vi "Begin.vi"(11 "Image Size":T1=enum."160x120") -> (0 "error out":errorcluster)   [LabVIEW 2012]
doc: "Called before other user functions, this VI is expected to open initial I/O refnums, load in file data, and do all program initialization. Notice that the <B>error out</B> terminal is simply used for data flow. Wiring it to other structures or subVIs ensures that this VI runs first."
uses:
  <vilib>/Rock Robotics/WPI/Camera/WPI_CameraImageSize.ctl
  <vilib>/Rock Robotics/SystemInterfaces/DIO/FPGA_DIOChannel.ctl
  <vilib>/Rock Robotics/WPI/CAN/Jaguar/SubVIs/WPI_CANJaguar_ControlMode.ctl
  <vilib>/Rock Robotics/WPI/Solenoid/WPI_SolenoidChannel.ctl
  <vilib>/Rock Robotics/SystemInterfaces/DIO/FPGA_DIORelayChannel.ctl
  <vilib>/Rock Robotics/WPI/Joystick/WPI_JoystickDeviceEnum.ctl
  <vilib>/Rock Robotics/SystemInterfaces/DIO/FPGA_DIOPWMChannel.ctl
  <vilib>/Rock Robotics/WPI/SafetyOutput/WPI_SafetyOutputConfigMenu.ctl
  <vilib>/Rock Robotics/WPI/Camera/WPI_CameraWhite Balance Values.ctl
  <vilib>/Rock Robotics/WPI/Camera/WPI_CameraExposure Values.ctl
  <vilib>/Rock Robotics/WPI/Camera/WPI_CameraFrameRate.ctl
  <vilib>/Rock Robotics/WPI/DriverStation/WPI_DriverStationRobotMode2.ctl
  <vilib>/Rock Robotics/WPI/MotorControl/WPI_MotorControlOpenCANJaguar.vi
  <vilib>/Rock Robotics/WPI/Solenoid/WPI_SolenoidOpenSingle.vi
  <vilib>/Rock Robotics/WPI/RobotDrive/WPI_RobotDriveOpen2MotorWithJaguar.vi
  Robot Global Data.vi
  <vilib>/Rock Robotics/WPI/Compressor/WPI_CompressorGetSetRefNum.vi
  <vilib>/Rock Robotics/WPI/CAN/Jaguar/SubVIs/WPI_CANJaguar_SpeedReference.ctl
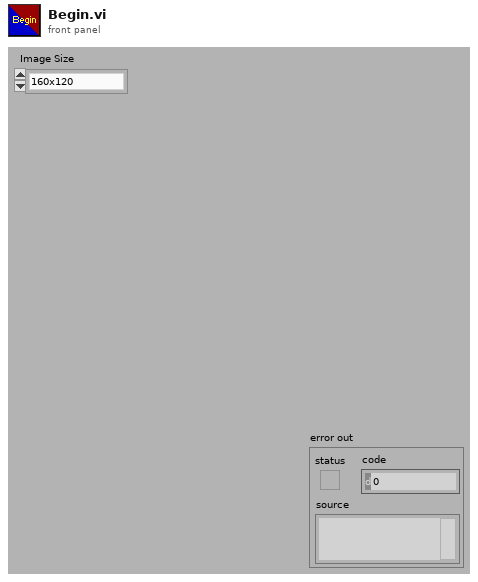
[diagram p1: front panel]
types:
  T1 = typedef "WPI_CameraImageSize.ctl" = enum16{"640x480", "320x240", "160x120"}
  T2 = typedef "WPI_DriverStationRobotMode2.ctl" = enum16{"Autonomous Disabled", "Autonomous Enabled", "Teleop Disabled", "Teleop Enabled", "Timeout", "Finish", "Test Disabled", "Test Enabled"}
  T3 = typedef "WPI_CameraFrameRate.ctl" = u32
  T4 = typedef "WPI_CameraExposure Values.ctl" = enum16{"Auto", "Flicker-free 50 Hz", "Flicker-free 60 Hz", "Hold current"}
  T5 = typedef "WPI_CameraWhite Balance Values.ctl" = enum16{"Auto", "Fixed indoor", "Fixed outdoor 1", "Fixed outdoor 2", "Fixed fluorescent 1", "Fixed fluorescent 2", "Hold current"}
  T6 = typedef "WPI_SafetyOutputConfigMenu.ctl" = enum16{"Enable", "Disable"}
  T7 = typedef "FPGA_DIOPWMChannel.ctl" = enum8{"PWM 1", "PWM 2", "PWM 3", "PWM 4", "PWM 5", "PWM 6", "PWM 7", "PWM 8", "PWM 9", "PWM 10", "Invalid"}
  T8 = typedef "WPI_JoystickDeviceEnum.ctl" = enum16{"USB 1", "USB 2", "USB 3", "USB 4", "Kinect 1", "Kinect 2"}
  T9 = typedef "FPGA_DIORelayChannel.ctl" = enum8{"Relay 1", "Relay 2", "Relay 3", "Relay 4", "Relay 5", "Relay 6", "Relay 7", "Relay 8", "Invalid"}
  T10 = typedef "WPI_SolenoidChannel.ctl" = enum8{"Solenoid 1", "Solenoid 2", "Solenoid 3", "Solenoid 4", "Solenoid 5", "Solenoid 6", "Solenoid 7", "Solenoid 8", "Invalid"}
  T11 = typedef "FPGA_DIOChannel.ctl" = enum8{"DIO 1", "DIO 2", "DIO 3", "DIO 4", "DIO 5", "DIO 6", "DIO 7", "DIO 8", "DIO 9", "DIO 10", "DIO 11", "DIO 12", "DIO 13", "DIO 14", "Invalid"}
  T12 = typedef "WPI_CANJaguar_ControlMode.ctl" = enum8{"Percent VBus", "Current", "Speed", "Position", "Voltage"}
  T13 = typedef "WPI_MotorControlDeviceRef.ctl" = cluster{"DeviceStatus":errorcluster, "Type":enum16{"PWM", "CAN"}, "PWM":cluster{"Digital Module":T14, "PWM Channel":T7, "DeadBand":T15}, "CAN":cluster{"Device Number":u8, "Control Mode":T12, "Semaphore":T16, "Max Vout":dbl}, "Invert":bool, "TransformRef":T17, "InvTransformRef":T17}
  T14 = typedef "FPGA_TypedefDigitalModule.ctl" = enum16{"Digital Module 1", "Digital Module 2"}
  T15 = typedef "WPI_PWMDeadband.ctl" = cluster{"Name":string, "maxPositivePwm":i32, "minPositivePwm":i32, "centerPwm":i32, "maxNegativePwm":i32, "minNegativePwm":i32, "angularRange":u16}
  T16 = typedef "Semaphore RefNum" = refnum<k1>
  T17 = typedef "WPI_PWMTransform_ConPane.ctl" = refnum<vi>
  T18 = typedef "WPI_CANJaguar_SpeedReference.ctl" = u8
  T19 = typedef "WPI_DigitalInputDevRef.ctl" = cluster{"DevStatus":errorcluster, "DIO Channel":T11, "Digital Module":T14}
  T20 = typedef "WPI_DigitalOutputDevRef.ctl" = cluster{"Digital Module":T14, "DIO Channel":T11, "DevStatus":errorcluster}
  T21 = typedef "WPI_JoystickDevRef.ctl" = cluster{"Device":T8}
  T22 = typedef "WPI_CompressorDevRef.ctl" = cluster{"DevStatus":errorcluster, "DigitalInputDevRef":T19, "RelayDevRef":T23}
  T23 = typedef "WPI_RelayDevRef.ctl" = cluster{"DevStatus":errorcluster, "Relay Channel":T9, "Digital Module":T14, "Relay Direction":T24}
  T24 = typedef "WPI_RelayDirection.ctl" = enum16{"Both directions", "Forward only", "Reverse only"}
  T25 = typedef "WPI_SolenoidDevRef.ctl" = cluster{"DevStatus":errorcluster, "Solenoid Module":T26, "Forward Solenoid Channel":T10, "Reverse Solenoid Channel":T10}
  T26 = typedef "FPGA_TypedefSolenoidModule.ctl" = enum16{"Solenoid Module 1", "Solenoid Module 2"}
  T27 = typedef "WPI_CameraDevRef.ctl" = cluster{"Camera Address":string, "CameraStatus":errorcluster, "Acquire Image Notifier":refnum<notifier>}
  T28 = typedef "WPI_RobotDriveDevRef.ctl" = cluster{"DevStatus":errorcluster, "Motors[]":T13[], "Square Inputs":bool, "Max Output":dbl, "Isochronous":bool}
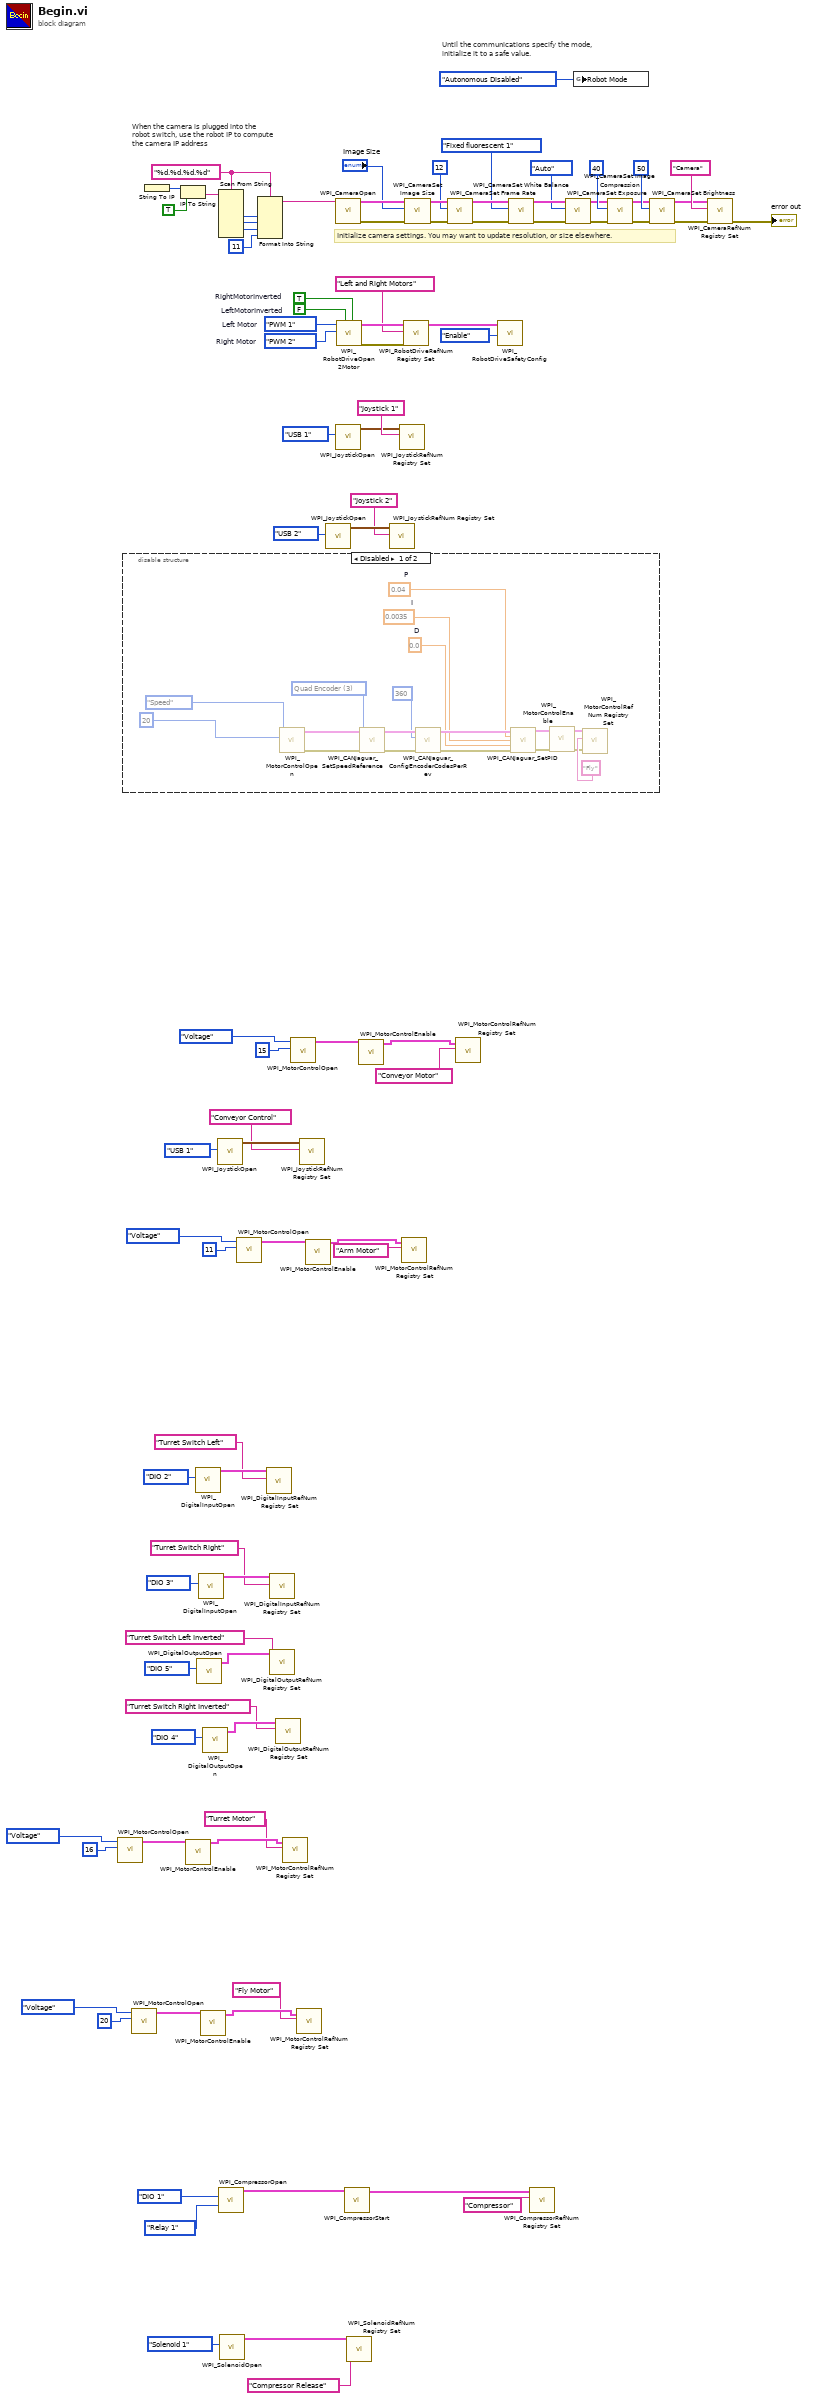
[diagram p0: block diagram]
diagram:
  w4 = "%d.%d.%d.%d" ("format string")
  w35 = FPGA_DIOPWMChannel."PWM 2"  # Right Motor
  w36 = FPGA_DIOPWMChannel."PWM 1"  # Left Motor
  w40 = FALSE  # LeftMotorInverted
  w41 = TRUE  # RightMotorInverted
  # "Until the communications specify the mode,\ninitialize it to a safe value."
  # "When the camera is plugged into the\nrobot switch, use the robot IP to compute\nthe camera IP address"
  # "Initialize camera settings. You may want to update resolution, or size elsewhere."
  n1 = call-poly <vilib>:"WPI_MotorControlOpen.vi"("Device Number"=u8 16, "Control Mode"=WPI_CANJaguar_ControlMode."Voltage") -> ("MotorControlDeviceRef"=w63:T13)  [unwired: 8 in, 1 out]
  n2 = disable-structure shown="Disabled" {
    frame Disabled {
      w93 = 0.0  # D
      w94 = 0.0035  # I
      w95 = 0.04  # P
      w99 = T18 3 items=["Encoder"=0, "Inv Encoder"=2, "Quad Encoder"=3, "None"=255] ("Speed Reference")
      n3 = call-poly <vilib>:"WPI_MotorControlOpen.vi"("Device Number"=u8 20, "Control Mode"=WPI_CANJaguar_ControlMode."Speed") -> ("error out"=w103:errorcluster, "MotorControlDeviceRef"=w102:T13)  [unwired: 8 in]
      n4 = call <vilib>:"WPI_CANJaguar_SetSpeedReference.vi"("error in (no error)"=w103, "Speed Reference"=w99, "CAN Jaguar Ref"=w102) -> ("error out"=w101:errorcluster, "CAN Jaguar Ref Out"=w100:T13)  [unwired: 7 in]
      n5 = call <vilib>:"WPI_CANJaguar_ConfigEncoderCodesPerRev.vi"("error in (no error)"=w101, "Encoder Codes Per Rev"=u16 360, "CAN Jaguar Ref"=w100) -> ("error out"=w96:errorcluster, "CAN Jaguar Ref Out"=w97:T13)  [unwired: 7 in]
      n6 = call <vilib>:"WPI_CANJaguar_SetPID.vi"("CAN Jaguar Ref"=w97, "P"=w95, "I"=w94, "D"=w93, "error in (no error)"=w96) -> ("CAN Jaguar Ref Out"=w92:T13, "error out"=w91:errorcluster)  [unwired: 9 in]
      n7 = call <vilib>:"WPI_MotorControlEnable.vi"("error in (no error)"=w91, "CAN Jaguar Ref"=w92) -> ("error out"=w104:errorcluster, "CAN Jaguar Ref Out"=w106:T13)  [unwired: 8 in]
      n8 = call <vilib>:"WPI_MotorControlRefNum Registry Set.vi"("error in (no error)"=w104, "refnum name"="Fly", "MotorControlDevRef"=w106) -> ()  [unwired: 7 in, 2 out]
    }
    frame Enabled {
    }
  }
  n9 = call-poly <vilib>:"WPI_MotorControlOpen.vi"("Device Number"=u8 20, "Control Mode"=WPI_CANJaguar_ControlMode."Voltage") -> ("MotorControlDeviceRef"=w58:T13)  [unwired: 8 in, 1 out]
  n10 = String To IP() -> (0:w11:u32)  [unwired: 1 in]
  n11 = IP To String(1:TRUE ("dot notation? (F)"), 2:w11) -> (0:w9:string)
  n12 = call <vilib>:"WPI_MotorControlEnable.vi"("CAN Jaguar Ref"=w63) -> ("CAN Jaguar Ref Out"=w64:T13)  [unwired: 9 in, 1 out]
  n13 = call <vilib>:"WPI_DigitalInputOpen.vi"("DIO Channel"=FPGA_DIOChannel."DIO 2") -> ("DigitalInputDevRef"=w76:T19)  [unwired: 9 in, 1 out]
  n14 = call <vilib>:"WPI_DigitalOutputOpen.vi"("DIO Channel"=FPGA_DIOChannel."DIO 5") -> ("DigitalOutputDevRef"=w70:T20)  [unwired: 9 in, 1 out]
  n15 = call <vilib>:"WPI_DigitalInputOpen.vi"("DIO Channel"=FPGA_DIOChannel."DIO 3") -> ("DigitalInputDevRef"=w73:T19)  [unwired: 9 in, 1 out]
  n16 = call <vilib>:"WPI_MotorControlEnable.vi"("CAN Jaguar Ref"=w58) -> ("CAN Jaguar Ref Out"=w59:T13)  [unwired: 9 in, 1 out]
  n17 = call <vilib>:"WPI_DigitalOutputOpen.vi"("DIO Channel"=FPGA_DIOChannel."DIO 4") -> ("DigitalOutputDevRef"=w67:T20)  [unwired: 9 in, 1 out]
  n18 = call <vilib>:"WPI_JoystickOpen.vi"("JoystickDevice"=WPI_JoystickDeviceEnum."USB 1") -> ("JoystickDevRef"=w84:T21)  [unwired: 10 in]
  n19 = Scan From String(format string=w4, input string=w9) -> (output 1=w8:i32, output 2=w7:i32, output 3=w6:i32)  [unwired: 7 in, 3 out]
  n20 = call <vilib>:"WPI_CompressorOpen.vi"("Pressure Switch DIO Channel"=FPGA_DIOChannel."DIO 1", "Relay Channel"=FPGA_DIORelayChannel."Relay 1") -> ("CompressorDevRef"=w49:T22)  [unwired: 12 in, 1 out]
  n21 = call-poly <vilib>:"WPI_SolenoidOpen.vi"("Solenoid Channel"=WPI_SolenoidChannel."Solenoid 1") -> ("SolenoidDevRef"=w52:T25)  [unwired: 9 in, 1 out]
  n22 = call-poly <vilib>:"WPI_MotorControlOpen.vi"("Device Number"=u8 11, "Control Mode"=WPI_CANJaguar_ControlMode."Voltage") -> ("MotorControlDeviceRef"=w80:T13)  [unwired: 8 in, 1 out]
  n23 = Format Into String(format string=w4, w8, w7, w6, 11 ("Compression")) -> (resulting string=w2:string)  [unwired: 2 in, 1 out]
  n24 = call <vilib>:"WPI_DigitalInputRefNum Registry Set.vi"("refnum name"="Turret Switch Left", "DigitalInputDevRef"=w76) -> ()  [unwired: 8 in, 2 out]
  n25 = call <vilib>:"WPI_DigitalInputRefNum Registry Set.vi"("refnum name"="Turret Switch Right", "DigitalInputDevRef"=w73) -> ()  [unwired: 8 in, 2 out]
  n26 = call <vilib>:"WPI_DigitalOutputRefNum Registry Set.vi"("refnum name"="Turret Switch Left Inverted", "DigitalOutputDevRef"=w70) -> ()  [unwired: 8 in, 2 out]
  n27 = call <vilib>:"WPI_DigitalOutputRefNum Registry Set.vi"("refnum name"="Turret Switch Right Inverted", "DigitalOutputDevRef"=w67) -> ()  [unwired: 8 in, 2 out]
  n28 = call <vilib>:"WPI_MotorControlRefNum Registry Set.vi"("refnum name"="Turret Motor", "MotorControlDevRef"=w64) -> ()  [unwired: 8 in, 2 out]
  n29 = call-poly <vilib>:"WPI_MotorControlOpen.vi"("Device Number"=u8 15, "Control Mode"=WPI_CANJaguar_ControlMode."Voltage") -> ("MotorControlDeviceRef"=w88:T13)  [unwired: 8 in, 1 out]
  n30 = call <vilib>:"WPI_MotorControlRefNum Registry Set.vi"("refnum name"="Fly Motor", "MotorControlDevRef"=w59) -> ()  [unwired: 8 in, 2 out]
  n31 = call <vilib>:"WPI_JoystickRefNum Registry Set.vi"("refnum name"="Conveyor Control", "JoystickDevRef"=w84) -> ()  [unwired: 8 in, 2 out]
  n32 = call <vilib>:"WPI_MotorControlEnable.vi"("CAN Jaguar Ref"=w80) -> ("CAN Jaguar Ref Out"=w81:T13)  [unwired: 9 in, 1 out]
  n33 = call <vilib>:"WPI_JoystickOpen.vi"("JoystickDevice"=WPI_JoystickDeviceEnum."USB 2") -> ("JoystickDevRef"=w44:T21)  [unwired: 10 in]
  n34 = call <vilib>:"WPI_CameraOpen.vi"("Camera Address"=w2) -> ("error out"=w23:errorcluster, "CameraDevRef"=w24:T27)  [unwired: 1 in, 8 out]
  n35 = call <vilib>:"WPI_JoystickOpen.vi"("JoystickDevice"=WPI_JoystickDeviceEnum."USB 1") -> ("JoystickDevRef"=w46:T21)  [unwired: 10 in]
  n36 = call-poly <vilib>:"WPI_RobotDriveOpen2Motor.vi"("Right Motor Inverted"=w41, "Left Motor Inverted"=w40, "Right Motor"=w35, "Left Motor"=w36) -> ("error out"=w37:errorcluster, "RobotDriveDevRef"=w39:T28)  [unwired: 1 in, 5 out]
  n37 = call <vilib>:"WPI_CompressorStart.vi"("CompressorDevRef"=w49) -> ("CompressorDevRef"=w48:T22)  [unwired: 9 in, 1 out]
  n38 = call <vilib>:"WPI_SolenoidRefNum Registry Set.vi"("refnum name"="Compressor Release", "SolenoidDevRef"=w52) -> ()  [unwired: 8 in, 2 out]
  n39 = call <vilib>:"WPI_MotorControlEnable.vi"("CAN Jaguar Ref"=w88) -> ("CAN Jaguar Ref Out"=w89:T13)  [unwired: 9 in, 1 out]
  n40 = call <vilib>:"WPI_JoystickRefNum Registry Set.vi"("refnum name"="Joystick 2", "JoystickDevRef"=w44) -> ()  [unwired: 8 in, 2 out]
  n41 = call <vilib>:"WPI_JoystickRefNum Registry Set.vi"("refnum name"="Joystick 1", "JoystickDevRef"=w46) -> ()  [unwired: 8 in, 2 out]
  n42 = call <vilib>:"WPI_MotorControlRefNum Registry Set.vi"("refnum name"="Arm Motor", "MotorControlDevRef"=w81) -> ()  [unwired: 8 in, 2 out]
  n43 = call <vilib>:"WPI_RobotDriveRefNum Registry Set.vi"("error in (no error)"=w37, "refnum name"="Left and Right Motors", "RobotDriveDevRef"=w39) -> ("RobotDriveDevRef"=w34:T28)  [unwired: 8 out]
  n44 = call <vilib>:"WPI_CameraSet Image Size.vi"("error in (no error)"=w23, "Image Size"="Image Size", "CameraDevRef"=w24) -> ("error out"=w22:errorcluster, "CameraDevRef Out"=w25:T27)  [unwired: 7 out]
  n45 = call <vilib>:"WPI_CameraSet Frame Rate.vi"("error in (no error)"=w22, "Frame Rate (fps)"=T3 12, "CameraDevRef"=w25) -> ("error out"=w21:errorcluster, "CameraDevRef Out"=w27:T27)  [unwired: 7 out]
  n46 = call <vilib>:"WPI_MotorControlRefNum Registry Set.vi"("refnum name"="Conveyor Motor", "MotorControlDevRef"=w89) -> ()  [unwired: 8 in, 2 out]
  n47 = call <vilib>:"WPI_RobotDriveSafetyConfig.vi"("mode"=WPI_SafetyOutputConfigMenu."Enable", "RobotDriveDevRef"=w34) -> ()  [unwired: 8 in, 2 out]
  n48 = call <vilib>:"WPI_CameraSet White Balance.vi"("error in (no error)"=w21, "White Balance"=WPI_CameraWhite_Balance_Values."Fixed fluorescent 1", "CameraDevRef"=w27) -> ("error out"=w20:errorcluster, "CameraDevRef Out"=w26:T27)  [unwired: 7 out]
  n49 = call <vilib>:"WPI_CompressorRefNum Registry Set.vi"("refnum name"="Compressor", "CompressorDevRef"=w48) -> ()  [unwired: 8 in, 2 out]
  n50 = call <vilib>:"WPI_CameraSet Exposure.vi"("error in (no error)"=w20, "Exposure"=WPI_CameraExposure_Values."Auto", "CameraDevRef"=w26) -> ("error out"=w19:errorcluster, "CameraDevRef Out"=w29:T27)  [unwired: 7 out]
  n51 = global write "Robot Global Data.vi" "Robot Mode"(WPI_DriverStationRobotMode2."Autonomous Disabled" ("Robot Mode")) -> ()
  n52 = call <vilib>:"WPI_CameraSet Image Compression.vi"("error in (no error)"=w19, "Compression"=40, "CameraDevRef"=w29) -> ("error out"=w18:errorcluster, "CameraDevRef Out"=w28:T27)  [unwired: 7 out]
  n53 = call <vilib>:"WPI_CameraSet Brightness.vi"("error in (no error)"=w18, "Brightness"=50, "CameraDevRef"=w28) -> ("error out"=w16:errorcluster, "CameraDevRef Out"=w17:T27)  [unwired: 7 out]
  n54 = call <vilib>:"WPI_CameraRefNum Registry Set.vi"("error in (no error)"=w16, "refnum name"="Camera", "CameraDevRef"=w17) -> ("error out"=→"error out":errorcluster)  [unwired: 8 out]
